vi "Write Store Value Msg.vi"(7 "Store Value Msg":refnum<class "Store Value Msg.lvclass">, 8 "error in (no error)":errorcluster, 11 "IED in":refnum<class "IED.lvclass">) -> (0 "error out":errorcluster, 3 "IED out":refnum<class "IED.lvclass">)   [LabVIEW 2015, in "IED Actor.lvlib" / "IED.lvclass"]
uses:
  IED.lvclass
  IED Messages/Store Value/Store Value Msg.lvclass
  IED.lvclass/IED.ctl
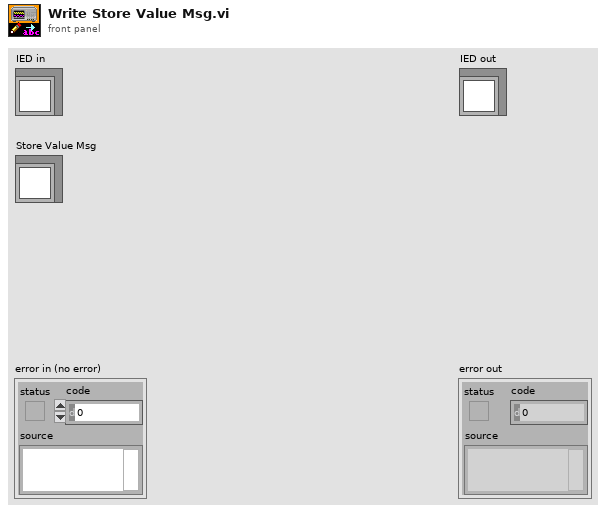
[diagram p1: front panel]
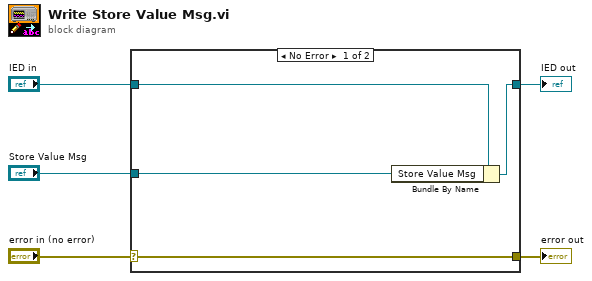
[diagram p0: block diagram]
diagram:
  n1 = case shown="No Error" "error in (no error)" {
    selector: "error in (no error)" -> [w9 w10]
    tunnel: [w9 w10] -> w4
    tunnel: [w7 w11] -> w2
    tunnel: "IED in" -> [w8 w11]
    tunnel: "Store Value Msg" -> [w6 _]
    frame No Error {
      n2 = Bundle By Name(cluster=w8, "Store Value Msg"=w6) -> (w7:refnum<class "IED.lvclass">)
    }
    frame Error {
    }
  }
  "error out" <- w4
  "IED out" <- w2
